vi "BLE_StopWatcher.vi"(0 ".NET Refnum in":refnum<k24>, 11 "error in (no error)":errorcluster) -> (4 ".NET Refnum out":refnum<k24>, 6 "StoptDeviceWatcher":string, 15 "error out":errorcluster)   [LabVIEW 2020]
uses:
  C:/Users/bharathi.t/Downloads/Bluetooth - Copy/Bluetooth/BLE/BLELib.dll
  BLELib.dll
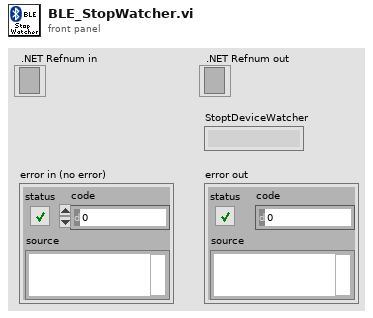
[diagram p1: front panel]
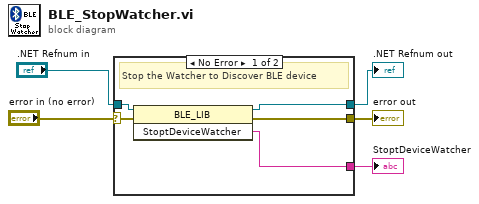
[diagram p0: block diagram]
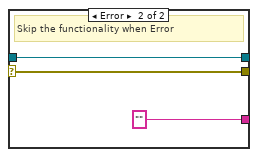
[diagram p2: hidden frame]
diagram:
  n1 = case shown="No Error" "error in (no error)" {
    selector: "error in (no error)" -> [w10 w12]
    tunnel: ".NET Refnum in" -> [w9 w13]
    tunnel: [w8 w13] -> w3
    tunnel: [w7 w12] -> w2
    tunnel: [w6 "" ("StoptDeviceWatcher")] -> w1
    frame No Error {
      # "Stop the Watcher to Discover BLE device"
      n2 = invoke class="BLE_LIB" method="StoptDeviceWatcher"(reference=w9, error in=w10) -> (reference out=w8:refnum<k24>, error out=w7:errorcluster, "StoptDeviceWatcher"=w6:string)  [unwired: 1 in]
    }
    frame Error {
      # "Skip the functionality when Error"
    }
  }
  ".NET Refnum out" <- w3
  "error out" <- w2
  "StoptDeviceWatcher" <- w1
